vi "initialise.vi"(8 "error in (no error)":errorcluster, 11 "ScanModeTS090821Circular2D in":refnum<class "ImagingModeTS090821Circular2D.lvclass">) -> (0 "error out":errorcluster, 3 "ScanModeTS090821Circular2D out":refnum<class "ImagingModeTS090821Circular2D.lvclass">)   [LabVIEW 2010, in "ImagingModeTS090821Circular2D.lvclass"]
doc: "The dynamic dispatch-version of this VI initalises the plug-in object by allocating and initalising any dynamic resources need."
uses:
  ImagingModeTS090821Circular2D.lvclass
  Display/GenericDisplay/GenericDisplay/GenericDisplay.lvclass
  common/classes/Image/Image/Image.lvclass
  DAQ/GenericDAQ/GenericDAQ/GenericDAQ.lvclass
  ScanHead/GenericScanHead/GenericScanHead/GenericScanHead.lvclass
  Stimulator/GenericStimulator/GenericStimulator/GenericStimulator.lvclass
  Instrument/GenericInstrument/GenericInstrument/GenericInstrument.lvclass
  <vilib>/vision/Image Controls.llb/IMAQ Image.ctl
  Analyser/GenericAnalyser/GenericAnalyser/GenericAnalyser.lvclass
  ImagingModeDL091001Scaffold/ImagingModeDL091001Scaffold/ImagingModeDL091001Scaffold.lvclass
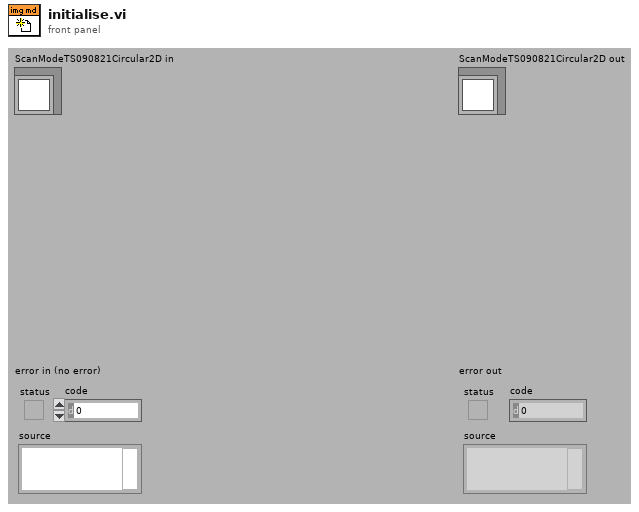
[diagram p1: front panel]
types:
  T1 = typedef "IMAQ Image.ctl" = refnum<image>
  T2 = typedef "Image Type" = u32
  T3 = typedef "controls_refs.ctl" = cluster{"scan start button":refnum<vi>, "tabs":cluster{"main":refnum<vi>, "settings":refnum<vi>}, "subpanels":cluster{"imagingMode":refnum<vi>, "scanHead":refnum<vi>, "display":refnum<vi>, "experimentController":refnum<vi>, "instrument":refnum<vi>, "stage":refnum<vi>, "stimulator":refnum<vi>, "dataCollection":refnum<vi>, "analyser":refnum<vi>, "daq":refnum<vi>, "imageAssembler":refnum<vi>}, "drop-downs":cluster{"run mode":refnum<vi>, "imagingMode":refnum<vi>, "experimentalController":refnum<vi>, "objective":refnum<vi>}, "status lights":cluster{"experimentController":refnum<vi>, "imagingMode":refnum<vi>, "scanHead":refnum<vi>, "daq":refnum<vi>, "imageAssembler":refnum<vi>, "dataCollection":refnum<vi>, "display":refnum<vi>, "analyser":refnum<vi>, "stage":refnum<vi>, "stimulator":refnum<vi>, "instrument":refnum<vi>}, "message":refnum<vi>, "stimulator enabled?":refnum<vi>, "saving":cluster{"data folder path":refnum<vi>, "file base name":refnum<vi>, "notebook":refnum<vi>}, "progress bar":refnum<vi>, "update icon":refnum<vi>, "title":refnum<vi>, "main vi":refnum<vi>, "user":refnum<vi>, "exit_button":refnum<vi>, "CPU usage %":refnum<vi>}
  T4 = typedef "plugin_specification.ctl" = cluster{"class path":string, "configuration":string, "label":string, "settings name":string}
  T5 = typedef "settings_specification_cluster.ctl" = cluster{"name":string, "label":string}
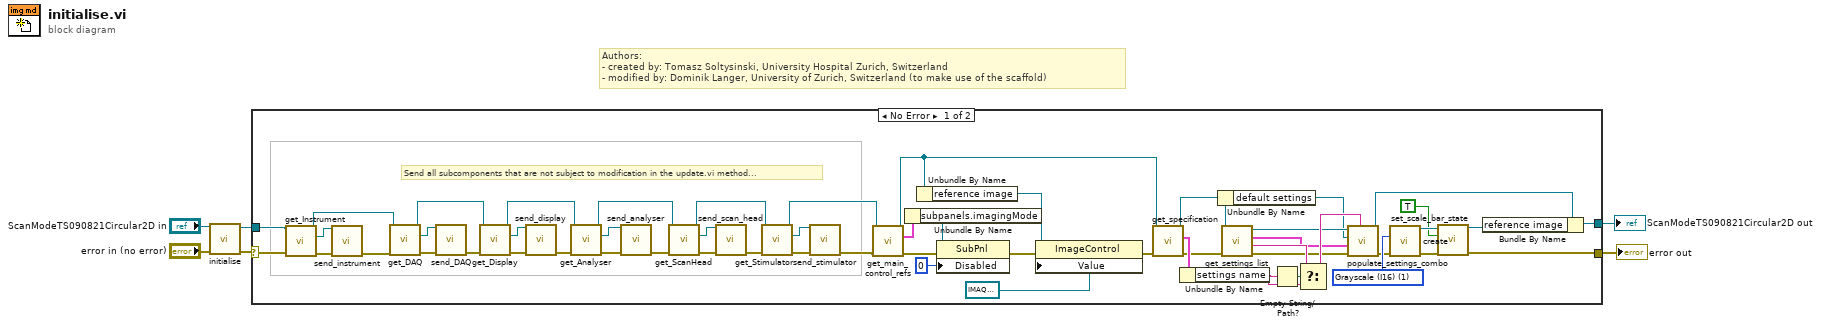
[diagram p0: block diagram]
diagram:
  # "Authors: \n- created by: Tomasz Soltysinski, University Hospital Zurich, Switzerland\n- modified by: Dominik Langer, University of Zurich, Switzerland (to make use of the scaffold)"
  n1 = call-parent "initialise.vi"("error in (no error)"="error in (no error)", "GenericPlugin in"="ScanModeTS090821Circular2D in") -> ("error out"=w4:errorcluster, "GenericPlugin out"=w1:refnum<class "ImagingModeTS090821Circular2D.lvclass">)  [unwired: 8 in]
  n2 = case shown="No Error" w4 {
    selector: w4 -> [w34 w62]
    tunnel: w1 -> [w33 w63]
    tunnel: [w28 w62] -> w2
    tunnel: [w7 w63] -> w3
    frame No Error {
      w57 = T2 1 items=["Grayscale (U8)", "Grayscale (I16)", "Grayscale (SGL)", "Complex (CSG)", "RGB (U32)", "HSL (U32)", "RGB (U64)", "Grayscale (U16)"] ("Image Type")
      # "Send all subcomponents that are not subject to modification in the update.vi method..."
      n3 = call-dynamic "get_Instrument.vi"("error in (no error)"=w34, "ScanModeDL090923Scaffold in"=w33) -> ("error out"=w35:errorcluster, "Instrument"=w36:refnum<class "GenericInstrument.lvclass">, "ScanModeDL090923Scaffold out"=w31:refnum<class "ImagingModeTS090821Circular2D.lvclass">)  [unwired: 4 in, 3 out]
      n4 = call-dynamic "send_instrument.vi"("error in (no error)"=w35, "GenericMicroscope in"=w36) -> ("error out"=w32:errorcluster)  [unwired: 8 in, 1 out]
      n5 = call-dynamic "get_DAQ.vi"("error in (no error)"=w32, "ScanModeDL090923Scaffold in"=w31) -> ("error out"=w56:errorcluster, "DAQ"=w55:refnum<class "GenericDAQ.lvclass">, "ScanModeDL090923Scaffold out"=w51:refnum<class "ImagingModeTS090821Circular2D.lvclass">)  [unwired: 4 in, 3 out]
      n6 = call-dynamic "send_DAQ.vi"("error in (no error)"=w56, "GenericDAQ in"=w55) -> ("error out"=w54:errorcluster)  [unwired: 8 in, 1 out]
      n7 = call-dynamic "get_Display.vi"("error in (no error)"=w54, "ScanModeDL090923Scaffold in"=w51) -> ("error out"=w53:errorcluster, "Display"=w52:refnum<class "GenericDisplay.lvclass">, "ScanModeDL090923Scaffold out"=w48:refnum<class "ImagingModeTS090821Circular2D.lvclass">)  [unwired: 4 in, 3 out]
      n8 = call-dynamic "send_display.vi"("error in (no error)"=w53, "GenericDisplay in"=w52) -> ("error out"=w49:errorcluster)  [unwired: 8 in, 1 out]
      n9 = call-dynamic "get_Analyser.vi"("error in (no error)"=w49, "ScanModeDL090923Scaffold in"=w48) -> ("error out"=w50:errorcluster, "Analyser"=w47:refnum<class "GenericAnalyser.lvclass">, "ScanModeDL090923Scaffold out"=w43:refnum<class "ImagingModeTS090821Circular2D.lvclass">)  [unwired: 4 in, 3 out]
      n10 = call-dynamic "send_analyser.vi"("error in (no error)"=w50, "GeneralAnalyser in"=w47) -> ("error out"=w45:errorcluster)  [unwired: 8 in, 1 out]
      n11 = call-dynamic "get_ScanHead.vi"("error in (no error)"=w45, "ScanModeDL090923Scaffold in"=w43) -> ("error out"=w46:errorcluster, "ScanHead"=w44:refnum<class "GenericScanHead.lvclass">, "ScanModeDL090923Scaffold out"=w41:refnum<class "ImagingModeTS090821Circular2D.lvclass">)  [unwired: 4 in, 3 out]
      n12 = call-dynamic "send_scan_head.vi"("error in (no error)"=w46, "GenericScanHead in"=w44) -> ("error out"=w42:errorcluster)  [unwired: 8 in, 1 out]
      n13 = call-dynamic "get_Stimulator.vi"("error in (no error)"=w42, "ScanModeDL090923Scaffold in"=w41) -> ("error out"=w40:errorcluster, "Stimulator"=w39:refnum<class "GenericStimulator.lvclass">, "ScanModeDL090923Scaffold out"=w37:refnum<class "ImagingModeTS090821Circular2D.lvclass">)  [unwired: 4 in, 3 out]
      n14 = call-dynamic "send_stimulator.vi"("error in (no error)"=w40, "GenericStimulator in"=w39) -> ("error out"=w38:errorcluster)  [unwired: 8 in, 1 out]
      n15 = call-dynamic "get_main_control_refs.vi"("error in (no error)"=w38, "GenericPlugin.lvclass in"=w37) -> ("error out"=w60:errorcluster, "control references"=w58:T3, "GenericPlugin.lvclass out"=w12:refnum<class "ImagingModeTS090821Circular2D.lvclass">)  [unwired: 7 out]
      n16 = Unbundle By Name(w58) -> ("subpanels.imagingMode"=w59:refnum<vi>)
      n17 = Unbundle By Name(w12) -> ("reference image"=w25:refnum<vi>)
      n18 = property class="SubPnl"(reference=w59, error in=w60, "Disabled"=u8 0) -> (error out=w23:errorcluster)  [unwired: 1 out]
      n19 = property class="ImageControl"(reference=w25, error in=w23, "Value"=T1 refnum ("Image")) -> (error out=w11:errorcluster)  [unwired: 1 out]
      n20 = call-dynamic "get_specification.vi"("error in (no error)"=w11, "GenericPlugin in"=w12) -> ("error out"=w16:errorcluster, "component specification"=w18:T4, "GenericPlugin out"=w17:refnum<class "ImagingModeTS090821Circular2D.lvclass">)  [unwired: 6 in, 1 out]
      n21 = Unbundle By Name(w18) -> ("settings name"=w20:string)
      n22 = Unbundle By Name(w17) -> ("default settings"=w9:refnum<vi>)
      n23 = call-dynamic "get_settings_list.vi"("error in (no error)"=w16, "ScanModeDL090923Scaffold in"=w17) -> ("error out"=w13:errorcluster, "default settings name"=w21:string, "combobox entries"=w15:T5[], "ScanModeDL090923Scaffold out"=w14:refnum<class "ImagingModeTS090821Circular2D.lvclass">)  [unwired: 6 in]
      n24 = Empty String/Path?(string/path=w20) -> (empty?=w19:bool)
      n25 = Select(t=w21, s=w19, f=w20) -> (s? t:f=w22:string)
      n26 = call-dynamic "populate_settings_combo.vi"("force settings"=w22, "error in (no error)"=w13, 9:w15, "combo box ref"=w9, "GenericPlugin in"=w14) -> ("error out"=w10:errorcluster, "GenericPlugin out"=w8:refnum<class "ImagingModeTS090821Circular2D.lvclass">)  [unwired: 5 in]
      n27 = call "create.vi"("error in (no error)"=w10, "Image Type"=w57) -> ("error out"=w30:errorcluster, "Image out"=w29:refnum<class "Image.lvclass">)  [unwired: 2 in, 6 out]
      n28 = call "set_scale_bar_state.vi"("error in (no error)"=w30, "enable?"=TRUE, "Image in"=w29) -> ("error out"=w28:errorcluster, "Image out"=w27:refnum<class "Image.lvclass">)  [unwired: 7 in]
      n29 = Bundle By Name(cluster=w8, "reference image"=w27) -> (w7:refnum<class "ImagingModeTS090821Circular2D.lvclass">)
    }
    frame Error {
    }
  }
  "error out" <- w2
  "ScanModeTS090821Circular2D out" <- w3
